vi "DriverVarianXGS-600.vi"(0 "VISA resource name":refnum<visa-resource-name>, 1 "Action":enum16{"Start", "Read", "Stop"}(ring), 2 "error in (no error)":errorcluster) -> (3 "Pressure connect?":bool, 4 "Pressure":dbl, 5 "VISA resource name out":refnum<visa-resource-name>, 6 "error out":errorcluster)   [LabVIEW 2019]
uses:
  <vilib>/Instr/_visa.llb/VISA Configure Serial Port (Instr).vi
panel:
  out "return count 3":u32
  out "return count 2":u32
  out "write buffer":string
  out "return count":u32
  out "error out 4":errorcluster
  out "error out 2":errorcluster
  out "read buffer":string
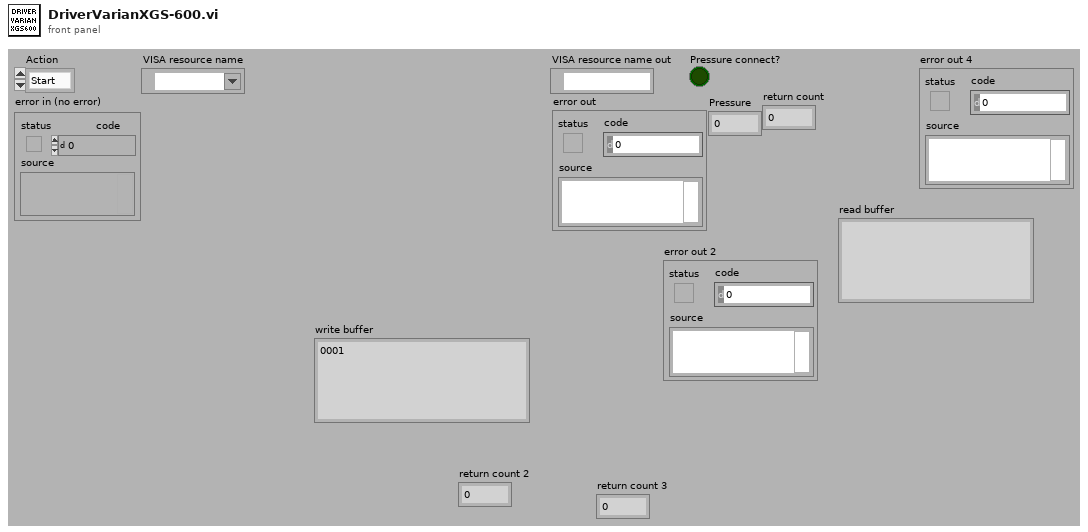
[diagram p1: front panel]
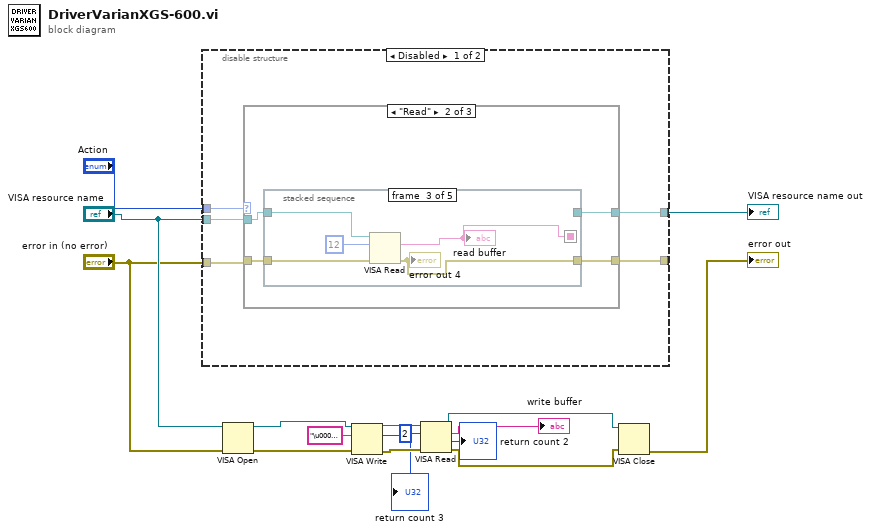
[diagram p0: block diagram]
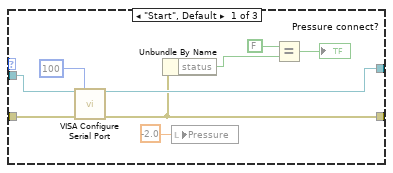
[diagram p2: hidden frame]
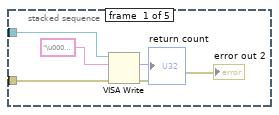
[diagram p3: hidden frame]
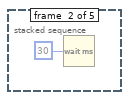
[diagram p4: hidden frame]
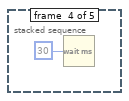
[diagram p5: hidden frame]
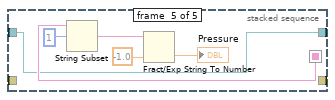
[diagram p6: hidden frame]
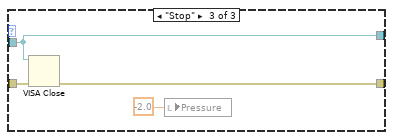
[diagram p7: hidden frame]
diagram:
  n1 = disable-structure shown="Disabled" {
    disable-tunnel: "Action" -> [w21 _]
    disable-tunnel: [w20 _] -> w15
    disable-tunnel: [w19 _] -> _
    disable-tunnel: "error in (no error)" -> [w18 _]
    disable-tunnel: "VISA resource name" -> [w17 _]
    frame Disabled {
      n2 = case shown="\"Read\"" w21 {
        tunnel: [w25 w32 w55] -> w19
        tunnel: [w29 w31 w54] -> w20
        tunnel: w18 -> [w28 w33 w56]
        tunnel: w17 -> [w27 w34 w54]
        frame "Start", Default {
          n3 = call-poly "VISA Configure Serial Port"("VISA resource name"=w27, "timeout (10sec)"=u32 100, "error in (no error)"=w28) -> ("VISA resource name out"=w29:refnum<visa-resource-name>, "error out"=w25:errorcluster)  [unwired: 11 in]
          n4 = Unbundle By Name(w25) -> ("status"=w24:bool)
          n5 = local write "Pressure"(-2.0 ("Pressure")) -> ()
          n6 = Equal?(x=FALSE, y=w24) -> (x = y?=→"Pressure connect?":bool)
        }
        frame "Read" {
          n7 = stacked-sequence {
            seq-local: [_ _ w42 _ _] -> [_ _ _ _ w52]
            tunnel: w34 -> [w38 _ w45 _ w47]
            tunnel: w33 -> [w39 _ w44 _ _]
            tunnel: [_ _ w41 _ _] -> w32
            tunnel: [_ _ _ _ w47] -> w31
            frame #0 {
              n8 = VISA Write(VISA resource name=w38, write buffer="\u0000\u000f", error in (no error)=w39) -> (return count=→"return count":u32, error out=→"error out 2":errorcluster)  [unwired: 1 out]
            }
            frame #1 {
              n9 = Wait (ms)(milliseconds to wait=u32 30) -> ()  [unwired: 1 out]
            }
            frame #2 {
              n10 = VISA Read(VISA resource name=w45, byte count=u32 12, error in (no error)=w44) -> (read buffer=w42:string, error out=w41:errorcluster)  [unwired: 2 out]
              "read buffer" <- w42
              "error out 4" <- w41
            }
            frame #3 {
              n11 = Wait (ms)(milliseconds to wait=u32 30) -> ()  [unwired: 1 out]
            }
            frame #4 {
              n12 = String Subset(string=w52, offset (0)=1) -> (substring=w50:string)  [unwired: 1 in]
              n13 = Fract/Exp String To Number(string=w50, default (0 dbl)=-1.0 ("default (0 DBL)")) -> (number=→"Pressure":dbl)  [unwired: 2 in, 1 out]
            }
          }
        }
        frame "Stop" {
          n14 = VISA Close(VISA resource name=w54, error in (no error)=w56) -> (error out=w55:errorcluster)
          n15 = local write "Pressure"(-2.0 ("Pressure")) -> ()
        }
      }
    }
    frame Enabled {
    }
  }
  "VISA resource name out" <- w15
  n16 = VISA Open(error in (no error)="error in (no error)", VISA resource name="VISA resource name") -> (VISA resource name=w6:refnum<visa-resource-name>, error out=w5:errorcluster)  [unwired: 3 in]
  n17 = VISA Write(VISA resource name=w6, write buffer="\u0000\u000f", error in (no error)=w5) -> (VISA resource name out=w12:refnum<visa-resource-name>, return count=→"return count 3":u32, error out=w11:errorcluster)
  n18 = VISA Read(VISA resource name=w12, byte count=u32 2, error in (no error)=w11) -> (VISA resource name out=w4:refnum<visa-resource-name>, read buffer=→"write buffer":string, return count=→"return count 2":u32, error out=w3:errorcluster)
  n19 = VISA Close(VISA resource name=w4, error in (no error)=w3) -> (error out=→"error out":errorcluster)
